vi "ReRouteAroundPolygon.vi"(2 "Desired Point Spacing (in)":dbl, 3 "AvoidancePolygon":T2, 4 "InputPath":T1[](array[typedef])) -> (0 "OutputPath":T1[](array[typedef]), 1 "PathChanged":bool)   [LabVIEW 2017]
uses:
  TypeDefs/Point2D.ctl
  TypeDefs/Polygon2D.ctl
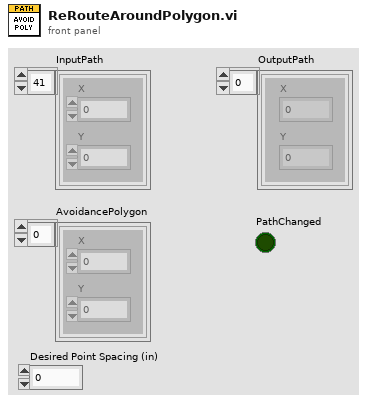
[diagram p1: front panel]
types:
  T1 = typedef "Point2D.ctl" = cluster{"X":dbl, "Y":dbl}
  T2 = typedef "Polygon2D.ctl" = T1[]
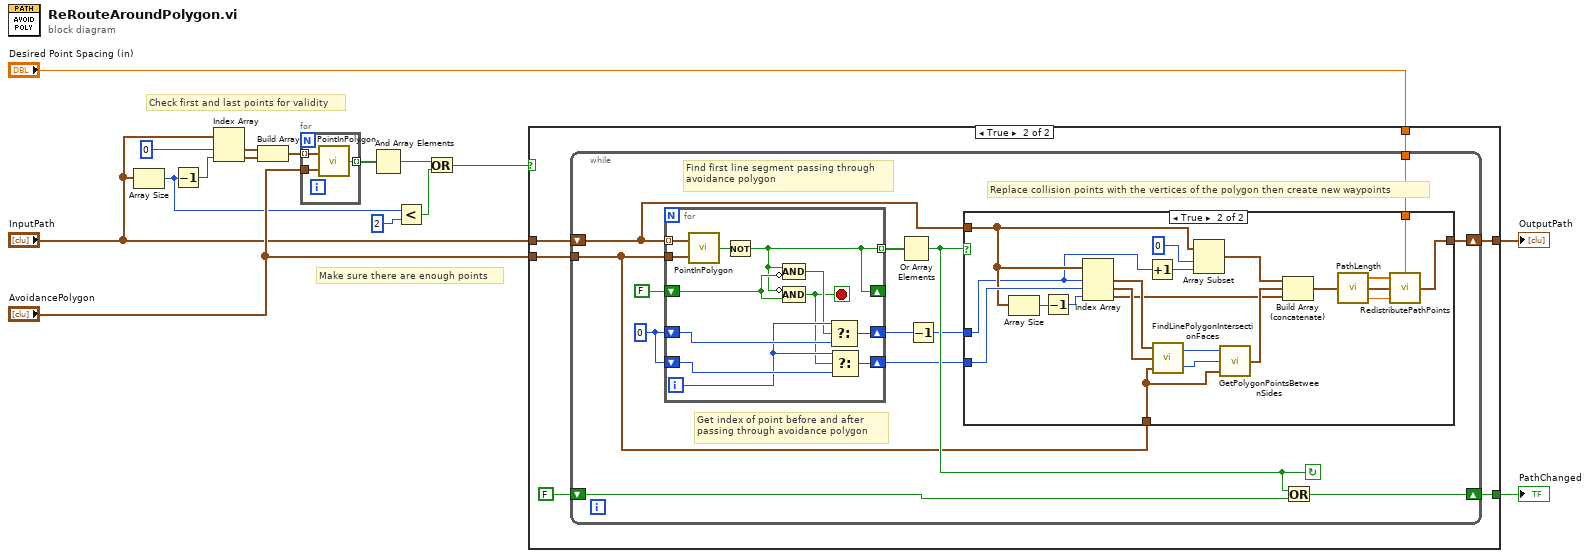
[diagram p0: block diagram]
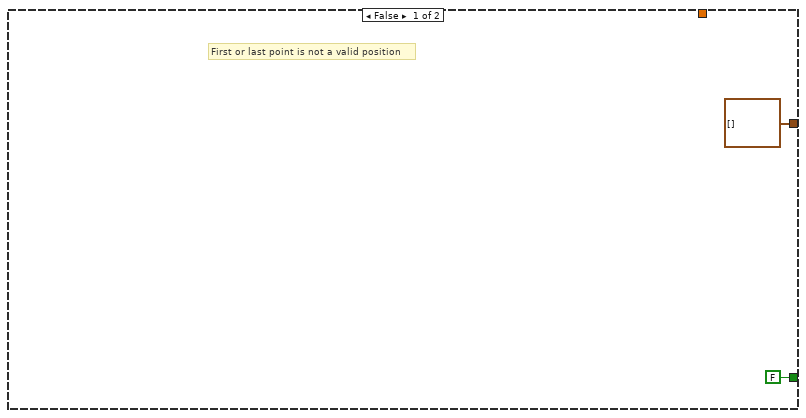
[diagram p2: hidden frame]
diagram:
  # "Make sure there are enough points"
  # "Check first and last points for validity"
  n1 = Array Size(array="InputPath") -> (size(s)=w2:i32)
  n2 = Decrement(x=w2) -> (x-1=w10:i32)
  n3 = Index Array(array="InputPath", index #1=0 ("index"), index #2=w10) -> (element #1=w9:T1, element #2=w8:T1)
  n4 = Build Array(w9, w8) -> (w7:T1[])
  n5 = for {
    tunnel: "AvoidancePolygon" -> [w19]
    tunnel: w7 -> [w18] mode=indexing
    tunnel: [w17] -> w6 mode=indexing
    n6 = call "PointInPolygon.vi"("Polygon"=w19, "2DPoint"=w18) -> ("InPolygon"=w17:bool)
  }
  n7 = And Array Elements(Boolean array=w6) -> (logical AND=w5:bool)
  n8 = Less?(x=w2, y=2) -> (x < y?=w3:bool)
  n9 = Or(x=w5, y=w3) -> (x .or. y?=w4:bool)
  n10 = case shown="True" w4 {
    tunnel: [T1[] [] ("InputPath") w27] -> w16
    tunnel: "Desired Point Spacing (in)" -> [_ w25]
    tunnel: [FALSE w24] -> w14
    tunnel: "AvoidancePolygon" -> [_ w23]
    tunnel: "InputPath" -> [_ w22]
    frame False {
      # "First or last point is not a valid position"
    }
    frame True {
      n11 = while {
        tunnel: w23 -> [w30]
        shift-right: [w34] -> w27
        shift-left: w22 -> [w28]
        shift-right: [w38] -> w24
        shift-left: FALSE -> [w37]
        tunnel: w25 -> [w29]
        stop <- w35 continue-if-true
        w36 = 0
        # "Replace collision points with the vertices of the polygon then create new waypoints"
        # "Get index of point before and after\npassing through avoidance polygon"
        # "Find first line segment passing through\navoidance polygon"
        n12 = for {
          tunnel: w28 -> [w64] mode=indexing
          tunnel: w30 -> [w74]
          tunnel: [w63] -> w40 mode=indexing
          shift-right: [w63] -> _
          shift-left: FALSE -> [w73]
          shift-right: [w71] -> w33
          shift-left: w36 -> [w70]
          shift-right: [w69] -> w31
          shift-left: w36 -> [w68]
          i -> [w67]
          stop <- w65 stop-if-true
          n13 = call "PointInPolygon.vi"("Polygon"=w74, "2DPoint"=w64) -> ("InPolygon"=w72:bool)
          n14 = Not(x=w72) -> (.not. x?=w63:bool)
          n15 = Compound Arithmetic op=AND(w63, invert w73) -> (w66:bool)
          n16 = Compound Arithmetic op=AND(invert w63, w73) -> (w65:bool)
          n17 = Select(t=w67, s=w66, f=w70) -> (s? t:f=w71:i32)
          n18 = Select(t=w67, s=w65, f=w68) -> (s? t:f=w69:i32)
        }
        n19 = Or Array Elements(Boolean array=w40) -> (logical OR=w35:bool)
        n20 = Decrement(x=w33) -> (x-1=w32:i32)
        n21 = case shown="True" w35 {
          tunnel: w28 -> [w41 w52]
          tunnel: [w41 w43] -> w34
          tunnel: w32 -> [_ w48]
          tunnel: w31 -> [_ w62]
          tunnel: w30 -> [_ w57]
          tunnel: w29 -> [_ w42]
          frame False {
            # "Path no longer goes through avoidance polygon"
          }
          frame True {
            n22 = Array Size(array=w52) -> (size(s)=w55:i32)
            n23 = Decrement(x=w55) -> (x-1=w54:i32)
            n24 = Index Array(array=w52, index #1=w48, index #2=w62, index #3=w54) -> (element #1=w61:T1, element #2=w60:T1, element #3=w53:T1)
            n25 = Increment(x=w48) -> (x+1=w49:i32)
            n26 = call "FindLinePolygonIntersectionFaces.vi"("Polygon"=w57, "ExitPoint"=w60, "EntryPoint"=w61) -> ("Exit Face"=w58:i32, "Entry Face"=w59:i32)
            n27 = Array Subset(array=w52, index=0, length=w49) -> (w50:T1[])
            n28 = call "GetPolygonPointsBetweenSides.vi"("Polygon"=w57, "LastSideIndex"=w58, "FirstSideIndex"=w59) -> ("PolygonVertices"=w56:T1[])
            n29 = Build Array (concatenate)(w50, w56, w53) -> (w47:T1[])
            n30 = call "PathLength.vi"("PathIn"=w47) -> ("Path Length"=w46:dbl, "PathOut"=w45:T1[], "IndexedPathLength"=w44:dbl[])  [unwired: 2 in]
            n31 = call "RedistributePathPoints.vi"("Desired Point Spacing (in)"=w42, "Path Length (in)"=w46, "PathIn"=w45, "IndexedPathLength"=w44) -> ("PathOut"=w43:T1[])
          }
        }
        n32 = Or(x=w35, y=w37) -> (x .or. y?=w38:bool)
      }
    }
  }
  "OutputPath" <- w16
  "PathChanged" <- w14
